vi "Check Loop Error.vi"(6 "Exit on Error? (F)":bool, 9 "Ignore Errors":i32[](array[numeric]), 10 "error to process":errorcluster) -> (2 "Error?":bool, 3 "channel":T1)   [LabVIEW 2019]
doc: "Check the 'error to process' to see if its code value matches any of the values in the 'Ignore Errors' array. If so, do nothing. If not, send an \"Error\" message containing the error data to the Message Handling Loop for further processing. If the \"Exit on Error?\" input is TRUE, send an \"Exit\" message to the Message Handling Loop instead."
uses:
  03.3 Queued Message Handler/support/Message Queue/Message Queue.lvlib
  Exercise 3-3/Producer Consumer (Events)/support/Message Queue/Message Cluster.ctl
  <extravilib>/ChannelInstances/Messenger-t'Message Queue.lvlib-Message Cluster.ctl'/))Channel.ctl
  <extravilib>/ChannelInstances/Messenger-t'Message Queue.lvlib-Message Cluster.ctl'.lvlib
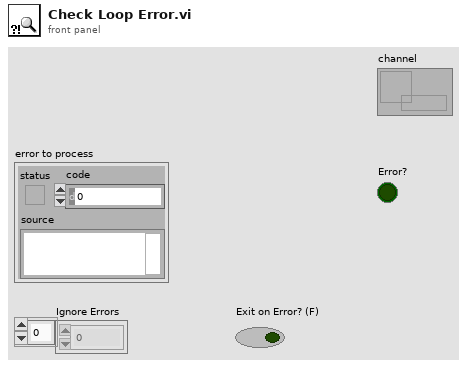
[diagram p1: front panel]
types:
  T1 = typedef "Messenger-t'Message Queue.lvlib-Message Cluster.ctl'.lvlib/))Channel.ctl" = refnum<queue>
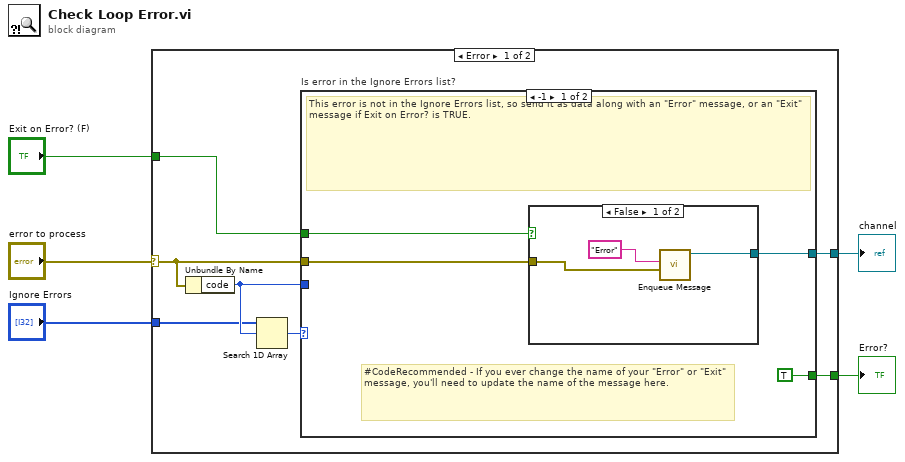
[diagram p0: block diagram]
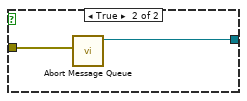
[diagram p2: hidden frame]
diagram:
  n1 = case shown="Error" "error to process" {
    selector: "error to process" -> [w9 _]
    tunnel: [w12 _] -> w3
    tunnel: "Ignore Errors" -> [w8 _]
    tunnel: [w7 _] -> w2
    tunnel: "Exit on Error? (F)" -> [w6 _]
    frame Error {
      n2 = Unbundle By Name(w9) -> ("code"=w10:i32)
      n3 = Search 1D Array(1D array=w8, element=w10) -> (index of element=w11:i32)  [unwired: 1 in]
      n4 = case "Is error in the Ignore Errors list?" shown="-1" w11 {
        tunnel: w9 -> [w15 _]
        tunnel: [w14 _] -> w12
        tunnel: w10 -> [_ _]
        tunnel: [TRUE _] -> w7
        tunnel: w6 -> [w13 _]
        frame -1 {
          # "#CodeRecommended - If you ever change the name of your \"Error\" or \"Exit\" message, you'll need to update the name of the message here."
          # "This error is not in the Ignore Errors list, so send it as data along with an \"Error\" message, or an \"Exit\" message if Exit on Error? is TRUE."
          n5 = case shown="False" w13 {
            tunnel: w15 -> [w19 w20]
            tunnel: [w18 w21] -> w14
            frame False {
              n6 = call "Enqueue Message.vi"("data (empty)"=w19, "message"="Error" ("Message")) -> ("channel"=w18:T1)  [unwired: 9 in]
            }
            frame True {
              n7 = call "Abort Message Queue.vi"("error to report"=w20) -> ("channel"=w21:T1)  [unwired: 10 in]
            }
          }
        }
        frame Default {
          # "This error is is in the Ignore Errors list, so do not send it for processing."
        }
      }
    }
    frame No Error {
      # "No error"
    }
  }
  "channel" <- w3
  "Error?" <- w2
